vi "Diff Tool.vi"(6 "Diff conflicts":T1[](array[typedef]), 7 "Message Queue":refnum<queue>, 8 "error in (no error)":errorcluster, 9 "roboRIO":path, 10 "Local":path, 11 "UI Data in":T2) -> (0 "error out":errorcluster, 3 "UI Data out":T2)   [LabVIEW 2018, in "Personalities Tool.lvlib"]
uses:
  Personalities Tool.lvlib
  Controls/QMH Data.ctl
  Controls/Personality Type.ctl
  Controls/roboRIO Connection Information.ctl
  Message Queue/Message Cluster.ctl
  Controls/Diff Key.ctl
  Configuration File.lvlibp/Configuration File.lvclass
  Message Queue/Enqueue Message (Single).vi
panel:
  in  "Select roboRIO":bool
  in  "Select Local":bool
  in  "Commit":bool
  in  "Open roboRIO":bool
  in  "Open Local":bool
  in  "Diff Options":T1[](array[typedef])
  # "Merge Conflicts Selector"
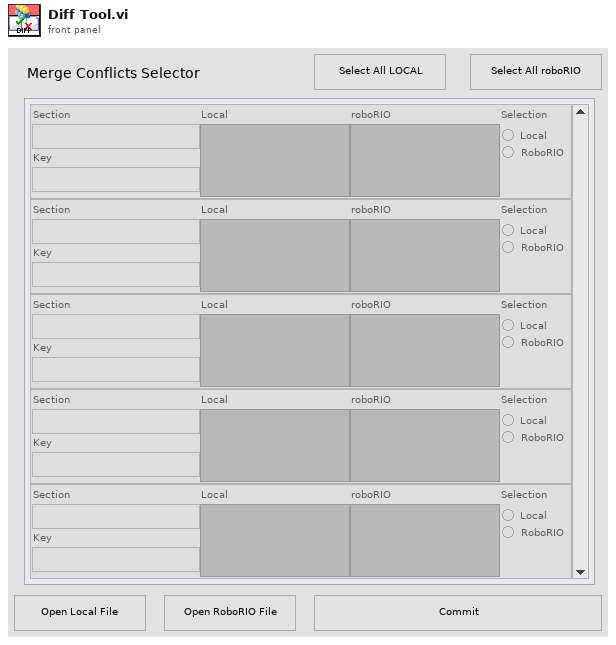
[diagram p1: front panel]
types:
  T1 = typedef "Personalities Tool.lvlib/Diff Key.ctl" = cluster{"Section":string, "Local":variant, "roboRIO":variant, "Selection":enum32{"Item 0", "Item 1"}, "Key":string}
  T2 = typedef "Personalities Tool.lvlib/QMH Data.ctl" = cluster{"Status":string, "Open Personality File Path":path, "File text":string, "Selected Personality":T3, "roboRIO Connection Information":T4, "VI reference":refnum<vi>, "Save personality locally reference":refnum<vi>, "File editor reference":refnum<vi>}
  T3 = typedef "Personalities Tool.lvlib/Personality Type.ctl" = cluster{"Valid personality?":bool, "Personality":string}
  T4 = typedef "Personalities Tool.lvlib/roboRIO Connection Information.ctl" = cluster{"Connected?":bool, "IP Address":string, "SN":string, "Personality":T3, "Name":string}
  T5 = enum32{"Invalid", "Standard", "Closed", "Hidden", "Minimized", "Maximized"}
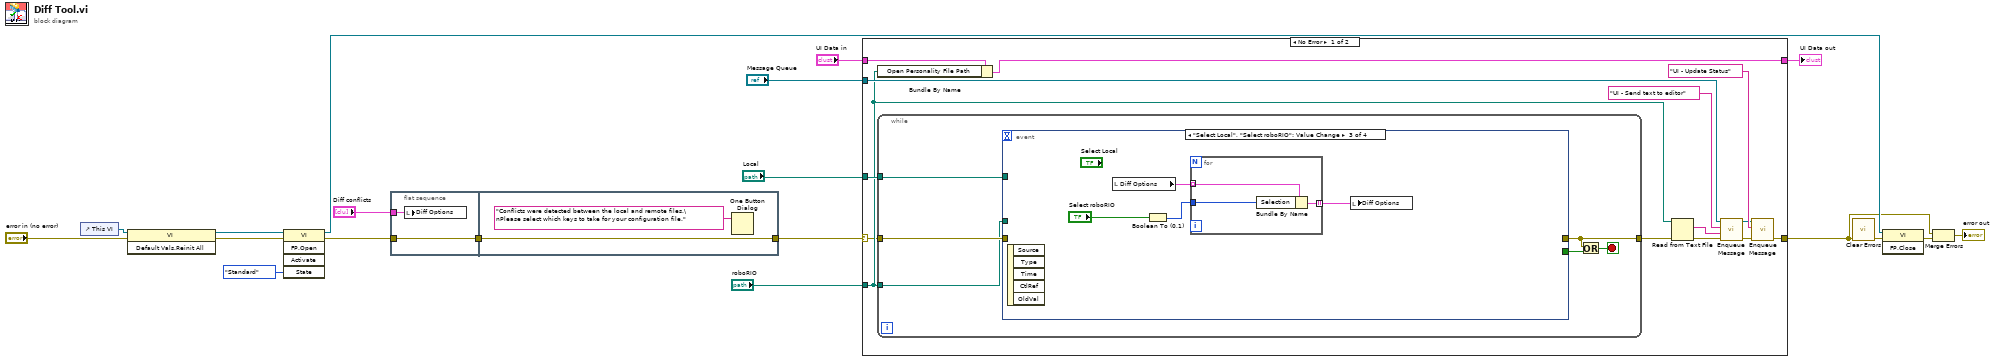
[diagram p0: block diagram]
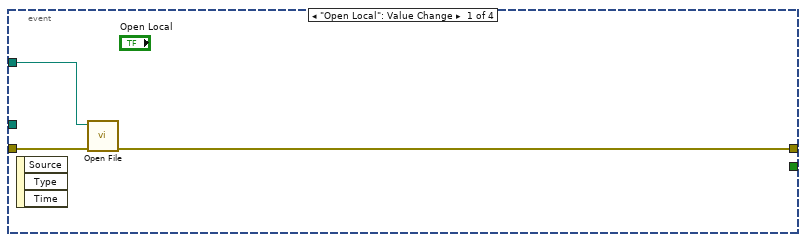
[diagram p2: hidden frame]
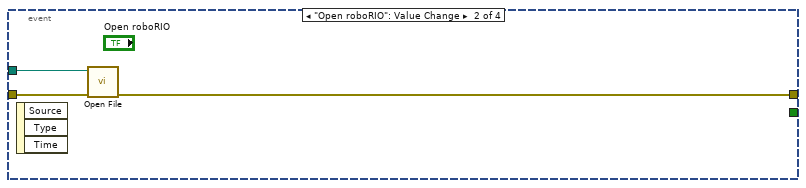
[diagram p3: hidden frame]
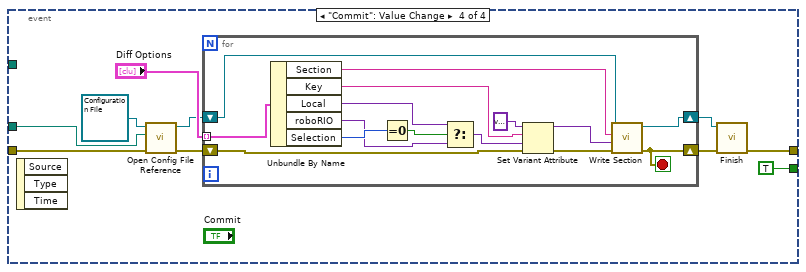
[diagram p4: hidden frame]
diagram:
  n1 = control-ref of="This VI"() -> (w13:refnum<vi>)
  n2 = invoke class="VI" method="Default Vals.Reinit All"(reference=w13, error in="error in (no error)") -> (reference out=w7:refnum<vi>, error out=w9:errorcluster)  [unwired: 1 in, 1 out]
  n3 = invoke class="VI" method="FP.Open"(reference=w7, error in=w9, "State"=T5."Standard") -> (reference out=w5:refnum<vi>, error out=w8:errorcluster)  [unwired: 2 in, 3 out]
  n4 = flat-sequence {
    tunnel: w8 -> [w21]
    tunnel: [w21] -> w12
    tunnel: "Diff conflicts" -> [w20]
    tunnel: [w22] -> w14
    tunnel: w12 -> [w22]
    frame #0 {
      n5 = local write "Diff Options"(w20) -> ()
    }
    frame #1 {
      n6 = One Button Dialog(message="Conflicts were detected between the local and remote files.\nPlease select which keys to take for your configuration file.") -> ()  [unwired: 1 in, 1 out]
    }
  }
  n7 = case shown="No Error" w14 {
    selector: w14 -> [w24 w83]
    tunnel: [w29 w83] -> w3
    tunnel: "Local" -> [w36 _]
    tunnel: "roboRIO" -> [w25 _]
    tunnel: "UI Data in" -> [w37 w82]
    tunnel: [w35 w82] -> w19
    tunnel: "Message Queue" -> [w28 _]
    frame No Error {
      n8 = Bundle By Name(cluster=w37, "Open Personality File Path"=w25) -> (w35:T2)
      n9 = while {
        tunnel: w24 -> [w43]
        tunnel: [w41] -> w30
        tunnel: w36 -> [w39]
        tunnel: w25 -> [w38]
        stop <- w42 stop-if-true
        n10 = event shown="[2] \"Select Local\", \"Select roboRIO\": Value Change" {
          selector: _ -> [_ _ _ _]
          dyn-events: _ -> [_ _ _ _]
          timeout: _ -> [_ _ _ _]
          tunnel: w43 -> [w46 w49 _ w60]
          tunnel: [w45 w48 _ w58] -> w41
          tunnel: [_ _ _ TRUE] -> w40
          tunnel: w39 -> [w44 _ _ _]
          tunnel: w38 -> [_ w47 _ w57]
          event "Open Local": Value Change {
            n11 = event-data() -> ()  [unwired: 1 in, 3 out]
            n12 = call "Open File.vi"("error in (no error)"=w46, "appended path"=w44) -> ("error out"=w45:errorcluster)  [unwired: 9 in]
          }
          event "Open roboRIO": Value Change {
            n13 = event-data() -> ()  [unwired: 1 in, 3 out]
            n14 = call "Open File.vi"("error in (no error)"=w49, "appended path"=w47) -> ("error out"=w48:errorcluster)  [unwired: 9 in]
          }
          event "Select Local", "Select roboRIO": Value Change {
            n15 = event-data() -> ()  [unwired: 1 in, 5 out]
            n16 = local read "Diff Options"() -> (w53:T1[])
            n17 = Boolean To (0,1)(Boolean="Select roboRIO") -> (0, 1=w50:i16)
            n18 = for {
              tunnel: w53 -> [w56] mode=indexing
              tunnel: [w55] -> w52 mode=indexing
              tunnel: w50 -> [w54]
              n19 = Bundle By Name(cluster=w56, "Selection"=w54) -> (w55:T1)
            }
            n20 = local write "Diff Options"(w52) -> ()
          }
          event "Commit": Value Change {
            n21 = event-data() -> ()  [unwired: 1 in, 3 out]
            n22 = call "Open Config File Reference.vi"("error in (no error)"=w60, "appended path"=w57, "Configuration File in"=refnum<class "Configuration File.lvclass"> refnum) -> ("error out"=w63:errorcluster, "Configuration File out"=w64:refnum<class "Configuration File.lvclass">)  [unwired: 7 in]
            n23 = for {
              tunnel: "Diff Options" -> [w81] mode=indexing
              shift-right: [w75] -> w62
              shift-left: w64 -> [w76]
              shift-right: [w67] -> w61
              shift-left: w63 -> [w71]
              stop <- w67 stop-if-true
              n24 = Unbundle By Name(w81) -> ("Section"=w74:string, "Key"=w73:string, "Local"=w78:variant, "roboRIO"=w77:variant, "Selection"=w80:enum32{"Item 0", "Item 1"})
              n25 = Equal To 0?(x=w80) -> (x = 0?=w79:bool)
              n26 = Select(t=w78, s=w79, f=w77) -> (s? t:f=w72:variant)
              n27 = Set Variant Attribute(Variant=variant ("variant"), name=w73, value=w72, error in=w71) -> (Variant out=w68:variant, error out=w70:errorcluster)  [unwired: 1 out]
              n28 = call-dynamic "Write Section.vi"("error in (no error)"=w70, "Section Data"=w68, "Section Name"=w74, "Configuration File in"=w76) -> ("error out"=w67:errorcluster, "Configuration File out"=w75:refnum<class "Configuration File.lvclass">)  [unwired: 6 in]
            }
            n29 = call-dynamic "Finish.vi"("error in (no error)"=w61, "Configuration File in"=w62) -> ("error out"=w58:errorcluster)  [unwired: 6 in, 3 out]
          }
        }
        n30 = Or(x=w41, y=w40) -> (x .or. y?=w42:bool)
      }
      n31 = Read from Text File(file (use dialog)=w25, error in=w30) -> (text=w26:string, error out=w27:errorcluster)  [unwired: 2 in, 2 out]
      n32 = call-poly "Enqueue Message.vi"("error in (no error)"=w27, "Message Data"=w26, "Message"="UI - Send text to editor", "Message Queue"=w28) -> ("error out"=w31:errorcluster, "dup Message Queue"=w32:refnum<queue>)  [unwired: 6 in]
      n33 = call-poly "Enqueue Message.vi"("error in (no error)"=w31, "Message"="UI - Update Status", "Message Queue"=w32) -> ("error out"=w29:errorcluster)  [unwired: 7 in, 1 out]
    }
    frame Error {
    }
  }
  "UI Data out" <- w19
  n34 = call <vilib>:"Clear Errors.vi"("error in (no error)"=w3) -> ("error out"=w4:errorcluster)  [unwired: 5 in, 1 out]
  n35 = invoke class="VI" method="FP.Close"(reference=w5, error in=w4) -> (error out=w1:errorcluster)  [unwired: 1 in, 2 out]
  n36 = Merge Errors(w3, w1) -> (→"error out":errorcluster)
